vi "RPC Method MeasurementService Measure Logic.vi"(8 "error in":errorcluster, 11 "gRPCid in":T1) -> (0 "error out":errorcluster)   [LabVIEW 2020, in "MeasurementLink Measurement Server.lvlib"]
uses:
  MeasurementLink Measurement Server.lvlib
  6e93e594-9b53-4a41-bad0-565312cbf1e4.vi
  <vilib>/gRPC/LabVIEW gRPC Library/grpc-lvsupport-release.lvlib
  <vilib>/gRPC/LabVIEW gRPC Library/Server API/typeDefs/gRPC Status Code.ctl
  c01dd925-8d21-4ce6-b452-e7218c44af5c.vi
  MeasurementLink Measurement Server Internal/RPC Service/MeasurementService/MeasurementService.lvclass
  MeasurementContext/MeasurementContext.lvclass
  <vilib>/gRPC/LabVIEW gRPC Library/Shared/grpcId.ctl
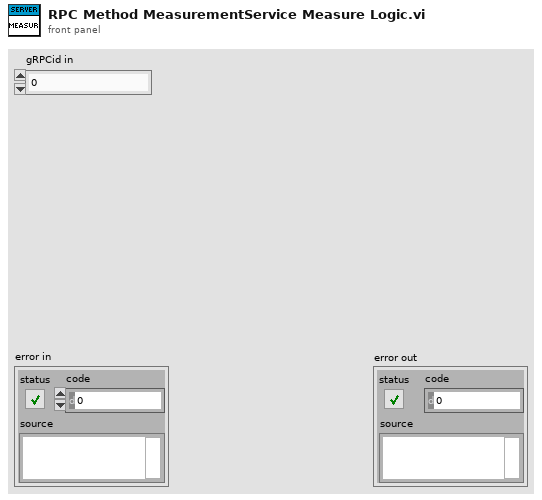
[diagram p1: front panel]
types:
  T1 = typedef "grpc-lvsupport-release.lvlib/grpcId.ctl" = u64
  T2 = typedef "MeasurementLink Measurement Server Internal.lvlib/ni_measurementlink_measurement_v1_MeasureRequest.ctl" = cluster{"configuration_parameters":T3, "pin_map_context":T4}
  T3 = typedef "MeasurementLink Measurement Server Internal.lvlib/google_protobuf_Any.ctl" = cluster{"type_url":string, "value":u8[]}
  T4 = typedef "MeasurementLink Measurement Server Internal.lvlib/ni_measurementlink_PinMapContext.ctl" = cluster{"pin_map_id":string, "sites":i32[]}
  T5 = typedef "grpc-lvsupport-release.lvlib/gRPC Status Code.ctl" = enum16{"OK", "CANCELLED", "UNKNOWN", "INVALID_ARGUMENT", "DEADLINE_EXCEEDED", "NOT_FOUND", "ALREADY_EXISTS", "PERMISSION_DENIED", "RESOURCE_EXHAUSTED", "FAILED_PRECONDITION", "ABORTED", "OUT_OF_RANGE", "UNIMPLEMENTED", "INTERNAL", "UNAVAILABLE", "DATA_LOSS", "UNAUTHENTICATED"}
  T6 = typedef "grpc-lvsupport-release.lvlib/Any.ctl" = cluster{"Type Url":string, "Bytes":u8[]}
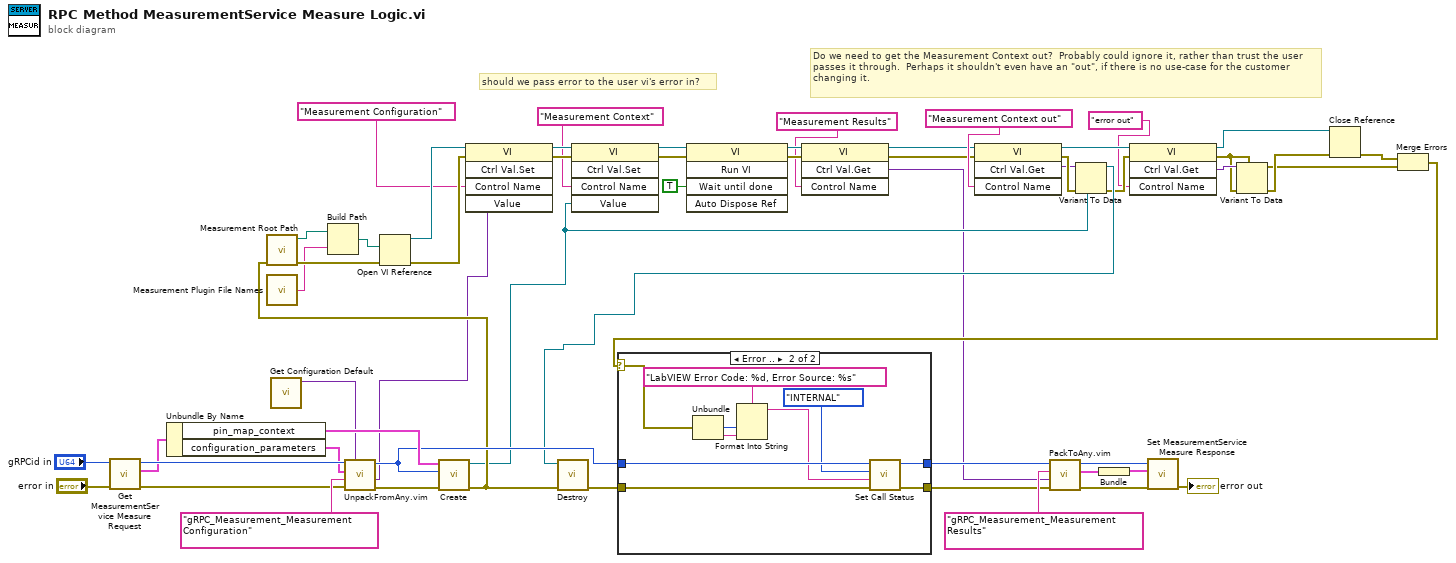
[diagram p0: block diagram]
diagram:
  # "should we pass error to the user vi's error in?"
  # "Do we need to get the Measurement Context out?  Probably could ignore it, rather than trust the user passes it through.  Perhaps it shouldn't even have an \"out\", if there is no use-case for the customer changing it."
  n1 = call "Get MeasurementService Measure Request.vi"("error in (no error)"="error in", "gRPCid in"="gRPCid in") -> ("error out"=w43:errorcluster, "Message Data"=w44:T2, "gRPCid out"=w45:T1)  [unwired: 7 in]
  n2 = Unbundle By Name(w44) -> ("pin_map_context"=w41:T4, "configuration_parameters"=w31:T3)
  n3 = call "Measurement Plugin File Names.vi"() -> ("Measurement Logic"=w34:string)  [unwired: 10 in, 5 out]
  n4 = call "Get Configuration Default.vi"() -> ("Measurement Configuration Default"=w30:variant)  [unwired: 10 in, 1 out]
  n5 = call "UnpackFromAny.vim"("Data Type"=w30, "error in"=w43, "Message Type"="gRPC_Measurement_Measurement Configuration", "Any"=w31, "gRPCid in"=w45) -> ("error out"=w42:errorcluster, "Unpacked Value"=w26:variant, "gRPCid out"=w39:u64)  [unwired: 4 in]
  n6 = call "Create.vi"("error in (no error)"=w42, "gRPC server call"=w39, "pin map context"=w41) -> ("error out"=w33:errorcluster, "MeasurementContext out"=w13:refnum<class "MeasurementContext.lvclass">)  [unwired: 7 in]
  n7 = call "Measurement Root Path.vi"("error in (no error)"=w33) -> ("error out"=w38:errorcluster, "Measurement Library Path out"=w37:path)  [unwired: 9 in]
  n8 = Build Path(base path=w37, name or relative path=w34) -> (appended path=w36:path)
  n9 = Open VI Reference(vi path=w36, error in (no error)=w38) -> (vi reference=w29:refnum<vi>, error out=w28:errorcluster)  [unwired: 4 in]
  n10 = invoke class="VI" method="Ctrl Val.Set"(reference=w29, error in=w28, "Control Name"="Measurement Configuration", "Value"=w26) -> (reference out=w25:refnum<vi>, error out=w24:errorcluster)  [unwired: 1 in, 3 out]
  n11 = invoke class="VI" method="Ctrl Val.Set"(reference=w25, error in=w24, "Control Name"="Measurement Context", "Value"=w13) -> (reference out=w21:refnum<vi>, error out=w22:errorcluster)  [unwired: 1 in, 3 out]
  n12 = invoke class="VI" method="Run VI"(reference=w21, error in=w22, "Wait until done"=TRUE ("Wait Until Done")) -> (reference out=w19:refnum<vi>, error out=w18:errorcluster)  [unwired: 2 in, 3 out]
  n13 = invoke class="VI" method="Ctrl Val.Get"(reference=w19, error in=w18, "Control Name"="Measurement Results") -> (reference out=w11:refnum<vi>, error out=w1:errorcluster, "Get Control Value Variant"=w2:variant)  [unwired: 1 in, 1 out]
  n14 = invoke class="VI" method="Ctrl Val.Get"(reference=w11, error in=w1, "Control Name"="Measurement Context out") -> (reference out=w10:refnum<vi>, error out=w15:errorcluster, "Get Control Value Variant"=w14:variant)  [unwired: 1 in, 1 out]
  n15 = Variant To Data(error in=w15, type=w13, Variant=w14) -> (data=w12:refnum<class "MeasurementContext.lvclass">, error out=w9:errorcluster)
  n16 = call-dynamic "Destroy.vi"("error in (no error)"=w33, "MeasurementContext in"=w12) -> ("error out"=w40:errorcluster)  [unwired: 9 in]
  n17 = invoke class="VI" method="Ctrl Val.Get"(reference=w10, error in=w9, "Control Name"="error out") -> (reference out=w6:refnum<vi>, error out=w5:errorcluster, "Get Control Value Variant"=w7:variant)  [unwired: 1 in, 1 out]
  n18 = Variant To Data(error in=w5, type=w5, Variant=w7) -> (data=w3:errorcluster, error out=w4:errorcluster)
  n19 = Close Reference(reference=w6, error in (no error)=w4) -> (error out=w35:errorcluster)
  n20 = Merge Errors(w35, w3) -> (w32:errorcluster)
  n21 = case shown="Error .." w32 {
    selector: w32 -> [_ w68]
    tunnel: w39 -> [w58 w67]
    tunnel: [w58 w66] -> w50
    tunnel: w40 -> [w57 w64]
    tunnel: [w57 w65] -> w49
    frame No Error {
    }
    frame Error {
      n22 = Unbundle(w68) -> ("code"=w62:i32, "source"=w61:string)  [unwired: 1 out]
      n23 = Format Into String(format string="LabVIEW Error Code: %d, Error Source: %s", w62, w61) -> (resulting string=w59:string)  [unwired: 2 in, 1 out]
      n24 = call <vilib>:"Set Call Status.vi"("error in"=w64, "Details"=w59, "Status Code"=gRPC_Status_Code."INTERNAL", "gRPCid in"=w67) -> ("error out"=w65:errorcluster, "gRPCid out"=w66:T1)  [unwired: 6 in]
    }
  }
  n25 = call "PackToAny.vim"("error in"=w49, "Data To Pack"=w2, "Message Type"="gRPC_Measurement_Measurement Results", "gRPCid in"=w50) -> ("error out"=w51:errorcluster, "Any"=w53:T6, "gRPCid out"=w54:u64)  [unwired: 5 in]
  n26 = Bundle("Any"=w53) -> (w52:cluster{"Any":T6})  [unwired: 1 in]
  n27 = call "Set MeasurementService Measure Response.vi"("error in (no error)"=w51, "Message Data"=w52, "gRPCid in"=w54) -> ("error out"=→"error out":errorcluster)  [unwired: 8 in]
